vi "Get Targets_Do.vi"(8 "error in (no error)":errorcluster, 11 "Dependency Source in":refnum<class "Dependency Source_VIPM.lvclass">) -> (0 "error out":errorcluster, 1 "Success?":bool, 2 "External Target Map":map{string, string}(c390), 3 "Internal Target Map":map{string, string}(c390), 4 "Unhandled Targets":string[](array[string]))   [LabVIEW 2019, in "Project.Dependencies Finder.lvlib" / "Dependency Source_VIPM.lvclass"]
doc: "Get internal and external targets for the dependency source.\n\nThis implementation gets VIPM targets."
uses:
  Dependency Source_VIPM.lvclass
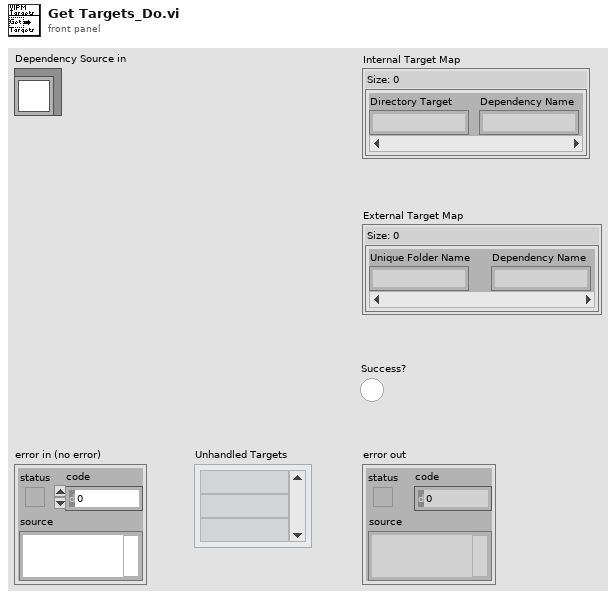
[diagram p1: front panel]
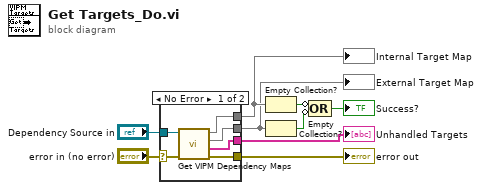
[diagram p0: block diagram]
diagram:
  n1 = case shown="No Error" "error in (no error)" {
    selector: "error in (no error)" -> [w15 w16]
    tunnel: [w14 w16] -> w9
    tunnel: [w12 _] -> w8
    tunnel: [w13 _] -> w7
    tunnel: [w11 _] -> w6
    tunnel: "Dependency Source in" -> [w10 _]
    frame No Error {
      n2 = call "Get VIPM Dependency Maps.vi"("error in"=w15, "Dependency Source_VIPM"=w10) -> ("error out"=w14:errorcluster, "Unmatched Packages"=w13:string[], "External Target Map"=w11:map{string, string}, "Internal Target Map"=w12:map{string, string})  [unwired: 6 in]
    }
    frame Error {
    }
  }
  "error out" <- w9
  "Internal Target Map" <- w8
  "External Target Map" <- w6
  "Unhandled Targets" <- w7
  n3 = Empty Collection?(1:w8) -> (0:w5:bool)
  n4 = Empty Collection?(1:w6) -> (0:w4:bool)
  n5 = Compound Arithmetic op=OR(invert w5, invert w4) -> (→"Success?":bool)
